vi "Dance.vi"(8 "error in (no error)":errorcluster) -> (0 "error out":errorcluster)   [LabVIEW 2017]
uses:
  fafe3425-db16-46cb-8cb9-fe815dfcc33b.vi
  2d8066bb-b678-43d1-aeb9-c388eb77b507.vi
  ee8a8f8c-2684-421b-9c4c-b7396520c37c.vi
  7c008b76-73c6-473b-866c-8ee7e2d2476b.vi
  24b98201-1d35-4c62-a4cd-72b9b23c5c63.vi
  b3b66bb1-3b43-4a8a-bd47-f6732c43c030.vi
  8d7e59c6-5f12-46c3-a736-9fcd407de2dd.vi
  6498f3fb-741d-44dc-a163-6ab251e79ac8.vi
  6a19dc3d-cbcb-4ebb-97bc-599d6f4eb225.vi
  e8e0193c-41b9-4e31-a30e-25b631857bbf.vi
  d00e3000-5418-4a74-97ce-523f092488f7.vi
  043285af-9ec3-490c-b740-177ba2c715b7.vi
  5b42c73d-f773-49b7-b1b4-47f0cf326e15.vi
panel:
  in  "Stop Button":bool
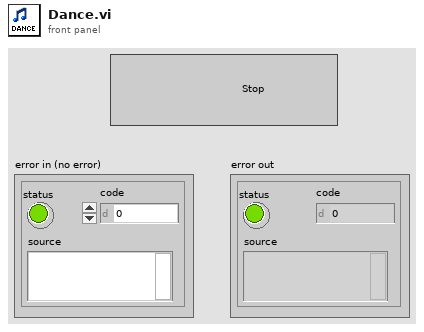
[diagram p1: front panel]
types:
  T1 = enum16{"off", "red", "green", "yellow", "blue", "pink", "cyan", "white"}
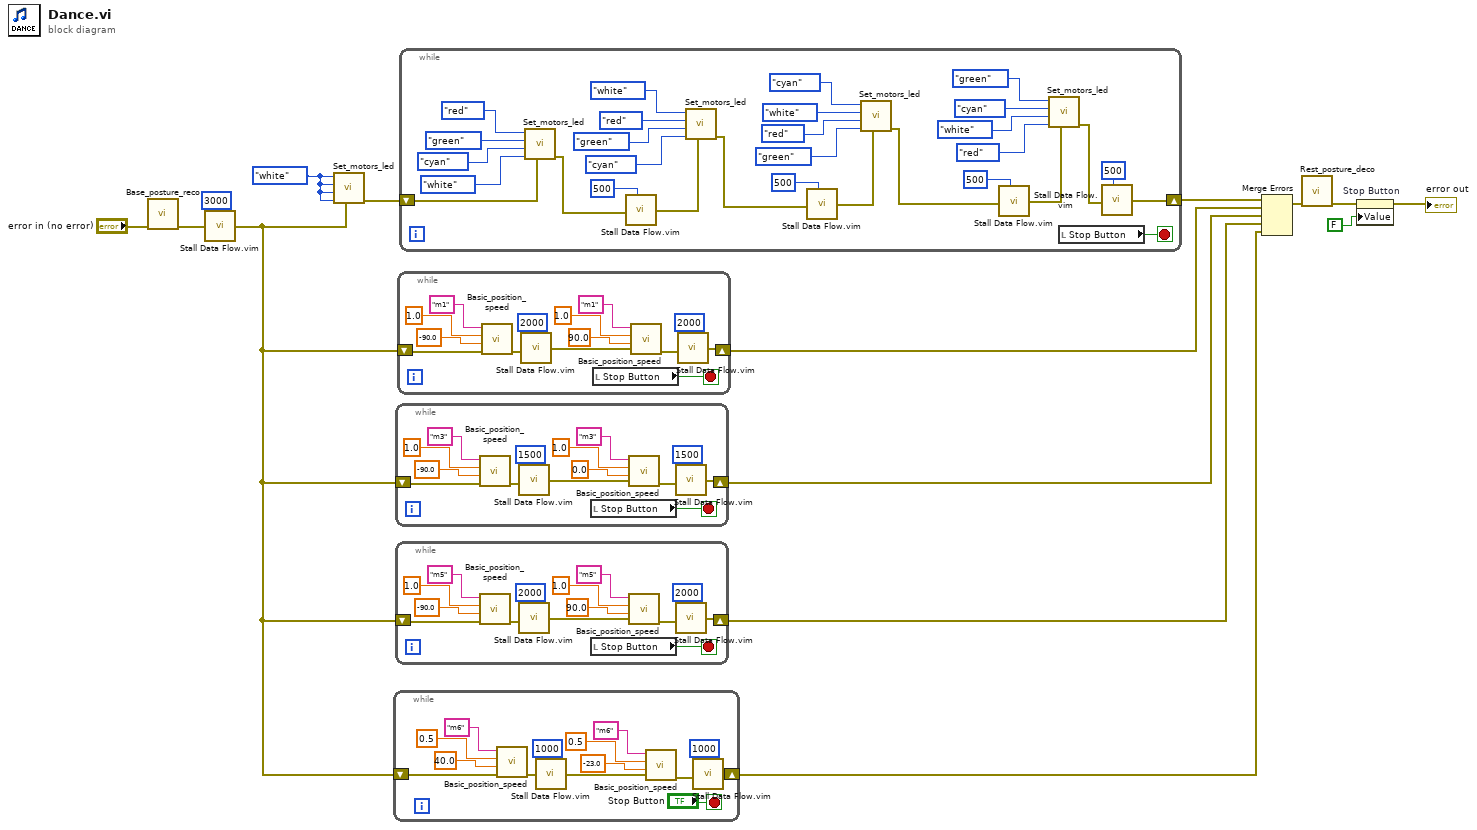
[diagram p0: block diagram]
diagram:
  w15 = T1."white" ("Color m2")
  n1 = call "Base_posture_reco.vi"("error in (no error)"="error in (no error)") -> ("error out"=w8:errorcluster)  [unwired: 10 in]
  n2 = call "Stall Data Flow.vim"("value in"=w8, "milliseconds to wait"=u32 3000) -> ("value out"=w1:errorcluster)  [unwired: 1 out]
  n3 = call "Set_motors_led.vi"("error in (no error)"=w1, "Color m6"=w15, "Color m5"=w15, "Color m3"=w15, "Color m2"=w15) -> ("error out"=w14:errorcluster)  [unwired: 6 in]
  n4 = while {
    shift-right: [w16] -> w2
    shift-left: w1 -> [w17]
    stop <- "Stop Button" stop-if-true
    n5 = call "Basic_position_speed.vi"("error in (no error)"=w17, "Position m?"=40.0, "Speed m?"=0.5, "m?"="m6") -> ("error out"=w21:errorcluster)  [unwired: 7 in]
    n6 = call "Stall Data Flow.vim"("value in"=w21, "milliseconds to wait"=u32 1000) -> ("value out"=w20:errorcluster)  [unwired: 1 out]
    n7 = call "Basic_position_speed.vi"("error in (no error)"=w20, "Position m?"=-23.0, "Speed m?"=0.5, "m?"="m6") -> ("error out"=w18:errorcluster)  [unwired: 7 in]
    n8 = call "Stall Data Flow.vim"("value in"=w18, "milliseconds to wait"=u32 1000) -> ("value out"=w16:errorcluster)  [unwired: 1 out]
  }
  n9 = while {
    shift-right: [w30] -> w4
    shift-left: w1 -> [w43]
    stop <- w33 stop-if-true
    n10 = call "Basic_position_speed.vi"("error in (no error)"=w43, "Position m?"=-90.0, "Speed m?"=1.0, "m?"="m3") -> ("error out"=w35:errorcluster)  [unwired: 7 in]
    n11 = call "Stall Data Flow.vim"("value in"=w35, "milliseconds to wait"=u32 1500) -> ("value out"=w34:errorcluster)  [unwired: 1 out]
    n12 = local read "Stop Button"() -> (w33:bool)
    n13 = call "Basic_position_speed.vi"("error in (no error)"=w34, "Position m?"=0.0, "Speed m?"=1.0, "m?"="m3") -> ("error out"=w31:errorcluster)  [unwired: 7 in]
    n14 = call "Stall Data Flow.vim"("value in"=w31, "milliseconds to wait"=u32 1500) -> ("value out"=w30:errorcluster)  [unwired: 1 out]
  }
  n15 = while {
    shift-right: [w44] -> w3
    shift-left: w1 -> [w57]
    stop <- w47 stop-if-true
    n16 = call "Basic_position_speed.vi"("error in (no error)"=w57, "Position m?"=-90.0, "Speed m?"=1.0, "m?"="m5") -> ("error out"=w49:errorcluster)  [unwired: 7 in]
    n17 = call "Stall Data Flow.vim"("value in"=w49, "milliseconds to wait"=u32 2000) -> ("value out"=w48:errorcluster)  [unwired: 1 out]
    n18 = local read "Stop Button"() -> (w47:bool)
    n19 = call "Basic_position_speed.vi"("error in (no error)"=w48, "Position m?"=90.0, "Speed m?"=1.0, "m?"="m5") -> ("error out"=w45:errorcluster)  [unwired: 7 in]
    n20 = call "Stall Data Flow.vim"("value in"=w45, "milliseconds to wait"=u32 2000) -> ("value out"=w44:errorcluster)  [unwired: 1 out]
  }
  n21 = while {
    shift-right: [w58] -> w11
    shift-left: w1 -> [w71]
    stop <- w61 stop-if-true
    n22 = call "Basic_position_speed.vi"("error in (no error)"=w71, "Position m?"=-90.0, "Speed m?"=1.0, "m?"="m1") -> ("error out"=w63:errorcluster)  [unwired: 7 in]
    n23 = call "Stall Data Flow.vim"("value in"=w63, "milliseconds to wait"=u32 2000) -> ("value out"=w62:errorcluster)  [unwired: 1 out]
    n24 = local read "Stop Button"() -> (w61:bool)
    n25 = call "Basic_position_speed.vi"("error in (no error)"=w62, "Position m?"=90.0, "Speed m?"=1.0, "m?"="m1") -> ("error out"=w59:errorcluster)  [unwired: 7 in]
    n26 = call "Stall Data Flow.vim"("value in"=w59, "milliseconds to wait"=u32 2000) -> ("value out"=w58:errorcluster)  [unwired: 1 out]
  }
  n27 = while {
    shift-right: [w74] -> w5
    shift-left: w14 -> [w101]
    stop <- w72 stop-if-true
    n28 = call "Set_motors_led.vi"("error in (no error)"=w101, "Color m6"=T1."white", "Color m5"=T1."cyan", "Color m3"=T1."green", "Color m2"=T1."red") -> ("error out"=w81:errorcluster)  [unwired: 6 in]
    n29 = call "Stall Data Flow.vim"("value in"=w81, "milliseconds to wait"=u32 500) -> ("value out"=w80:errorcluster)  [unwired: 1 out]
    n30 = call "Set_motors_led.vi"("error in (no error)"=w80, "Color m6"=T1."cyan", "Color m5"=T1."green", "Color m3"=T1."red", "Color m2"=T1."white") -> ("error out"=w79:errorcluster)  [unwired: 6 in]
    n31 = call "Stall Data Flow.vim"("value in"=w79, "milliseconds to wait"=u32 500) -> ("value out"=w78:errorcluster)  [unwired: 1 out]
    n32 = call "Set_motors_led.vi"("error in (no error)"=w78, "Color m6"=T1."green", "Color m5"=T1."red", "Color m3"=T1."white", "Color m2"=T1."cyan") -> ("error out"=w77:errorcluster)  [unwired: 6 in]
    n33 = call "Stall Data Flow.vim"("value in"=w77, "milliseconds to wait"=u32 500) -> ("value out"=w76:errorcluster)  [unwired: 1 out]
    n34 = call "Set_motors_led.vi"("error in (no error)"=w76, "Color m6"=T1."red", "Color m5"=T1."white", "Color m3"=T1."cyan", "Color m2"=T1."green") -> ("error out"=w73:errorcluster)  [unwired: 6 in]
    n35 = local read "Stop Button"() -> (w72:bool)
    n36 = call "Stall Data Flow.vim"("value in"=w73, "milliseconds to wait"=u32 500) -> ("value out"=w74:errorcluster)  [unwired: 1 out]
  }
  n37 = Merge Errors(w5, w11, w4, w3, w2) -> (w6:errorcluster)
  n38 = call "Rest_posture_deco.vi"("error in (no error)"=w6) -> ("error out"=w7:errorcluster)  [unwired: 10 in]
  n39 = property on="Stop Button" class="Bool (strict)"(error in=w7, "Value"=FALSE ("Stop Button")) -> (error out=→"error out":errorcluster)  [unwired: 1 in, 1 out]
